vi "Close.vi"(8 "error in (no error)":errorcluster, 11 "Abstract_Powermeter in":refnum<class "Abstract_Powermeter.lvclass">) -> (0 "error out":errorcluster, 3 "Abstract_Powermeter out":refnum<class "Abstract_Powermeter.lvclass">)   [LabVIEW 2020, in "Abstract_Powermeter.lvclass"]
uses:
  <instrlib>/Classes/Powermeter/Abstract/Abstract_Powermeter.lvclass
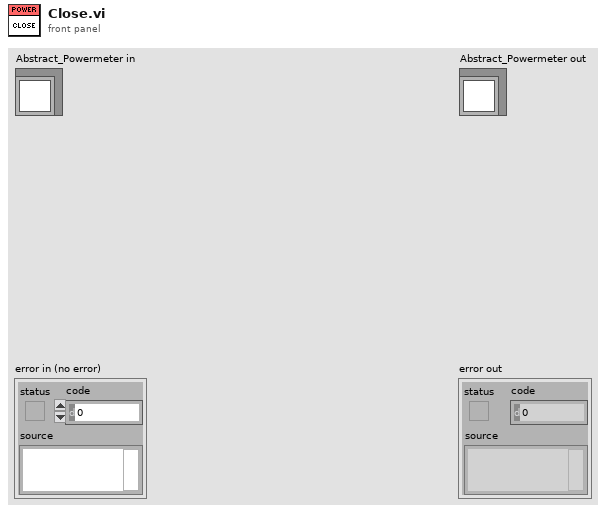
[diagram p1: front panel]
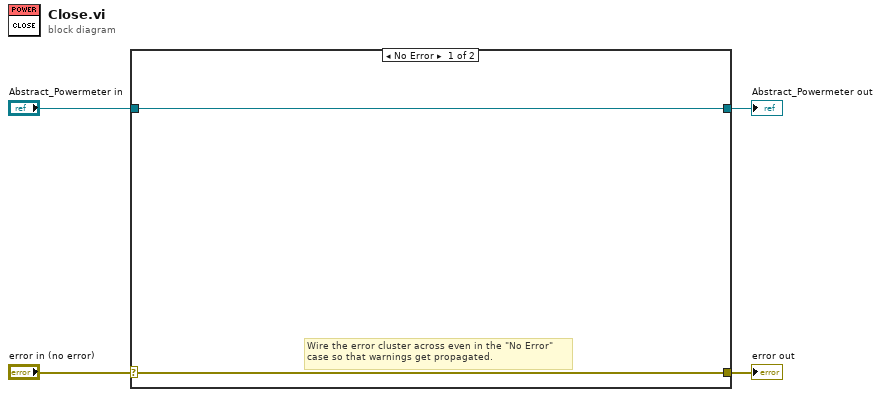
[diagram p0: block diagram]
diagram:
  n1 = case shown="No Error" "error in (no error)" {
    selector: "error in (no error)" -> [w5 w8]
    tunnel: [w5 w8] -> w3
    tunnel: [w6 w7] -> w1
    tunnel: "Abstract_Powermeter in" -> [w6 w7]
    frame No Error {
      # "Wire the error cluster across even in the \"No Error\"\ncase so that warnings get propagated."
    }
    frame Error {
    }
  }
  "error out" <- w3
  "Abstract_Powermeter out" <- w1
